vi "Write to Hardware.vi"(7 "Valid Triggers":bool, 8 "error in":errorcluster, 9 "Trigger Values":dbl[](array[numeric]), 10 "Values in":dbl[](array[numeric]), 11 "Rx UDP Execution Unit in":refnum<class "Rx UDP Execution Unit.lvclass">) -> (0 "error out":errorcluster, 1 "Trigger Values out":dbl[](array[numeric]), 2 "Values out":dbl[](array[numeric]), 3 "Rx UDP Execution Unit out":refnum<class "Rx UDP Execution Unit.lvclass">)   [LabVIEW 2020, in "AIM ARINC 664 Engine.lvlib" / "Implementation.lvlib" / "Rx UDP Execution Unit.lvclass"]
uses:
  Rx UDP Execution Unit.lvclass
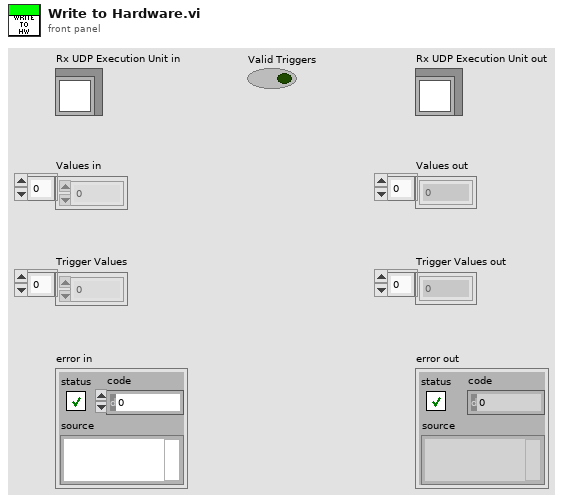
[diagram p1: front panel]
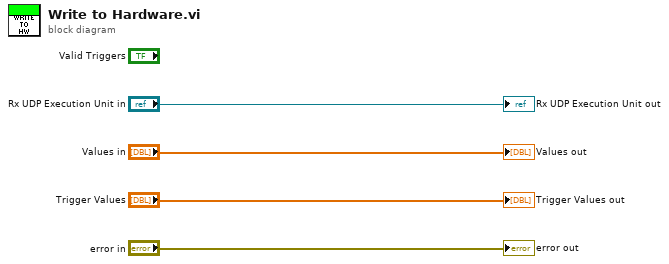
[diagram p0: block diagram]
diagram:
  "error out" <- "error in"
  "Rx UDP Execution Unit out" <- "Rx UDP Execution Unit in"
  "Values out" <- "Values in"
  "Trigger Values out" <- "Trigger Values"
